vi "Write Head and Air State.vi"(10 "Head and Air actions":T1, 11 "Temperature Control in":refnum<class "Temperature Control.lvclass">) -> (3 "Temperature Control out":refnum<class "Temperature Control.lvclass">)   [LabVIEW 2020, in "Temperature Control.lvclass"]
uses:
  Temperature Control.lvclass
  Controls/Head and Air actions.ctl
  Temperature Control.lvclass/Temperature Control.ctl
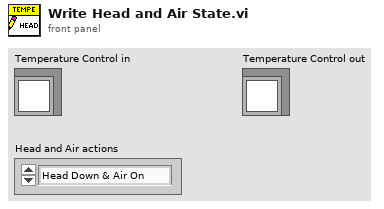
[diagram p1: front panel]
types:
  T1 = typedef "Temperature Control.lvclass/Head and Air actions.ctl" = enum16{"Head Down & Air On", "Head Up & Air Off", "Head Down", "Head Up", "Air On", "Air Off", "Compressor On", "Compressor Off"}
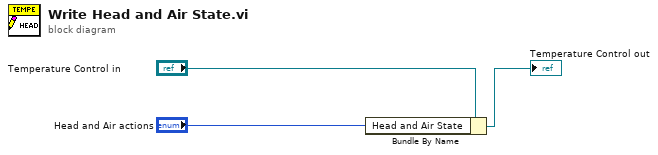
[diagram p0: block diagram]
diagram:
  n1 = Bundle By Name(cluster="Temperature Control in", "Head and Air State"="Head and Air actions") -> (→"Temperature Control out":refnum<class "Temperature Control.lvclass">)
